vi "Write WorkDir.vi"(8 "error in (no error)":errorcluster, 10 "WorkDir":path=path "D:/Test XDisplay images", 11 "Camera Dir Dialog in":refnum<class "Camera Dir Dialog.lvclass">) -> (0 "error out":errorcluster, 3 "Camera Dir Dialog out":refnum<class "Camera Dir Dialog.lvclass">)   [LabVIEW 2014, in "Camera Dir Dialog.lvlib" / "Camera Dir Dialog.lvclass"]
uses:
  Camera Dir Dialog.lvclass
  Camera Dir Dialog.lvclass/Camera Dir Dialog.ctl
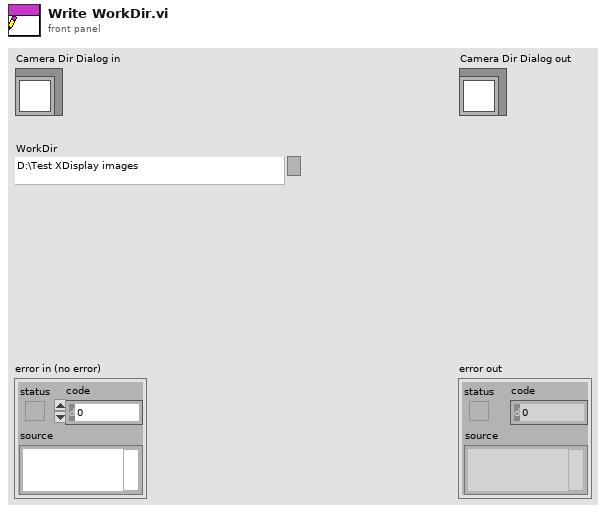
[diagram p1: front panel]
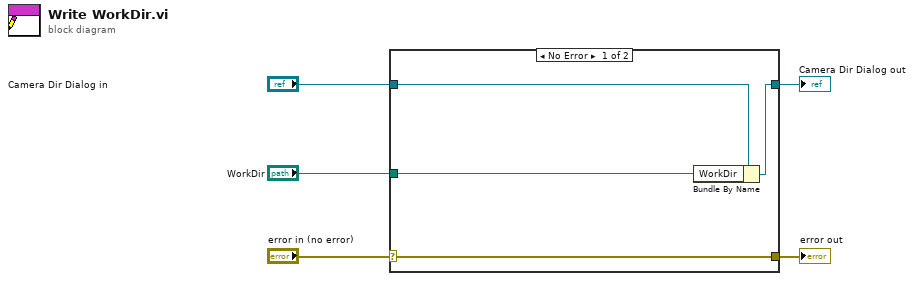
[diagram p0: block diagram]
diagram:
  n1 = case shown="No Error" "error in (no error)" {
    selector: "error in (no error)" -> [w9 w10]
    tunnel: [w9 w10] -> w4
    tunnel: [w7 w11] -> w2
    tunnel: "Camera Dir Dialog in" -> [w8 w11]
    tunnel: "WorkDir" -> [w6 _]
    frame No Error {
      n2 = Bundle By Name(cluster=w8, "WorkDir"=w6) -> (w7:refnum<class "Camera Dir Dialog.lvclass">)
    }
    frame Error {
    }
  }
  "error out" <- w4
  "Camera Dir Dialog out" <- w2
